vi "Tree.vi"   [LabVIEW 2019, in "DAQmx.lvclass"]
uses:
  DAQmx.lvclass
  C:/Program Files/National Instruments/LabVIEW 2019/vi.lib/JKI/JKI SMO/SMO/SMO.lvclass
  <vilib>/JKI/JKI SMO/SMO/SMO.lvclass
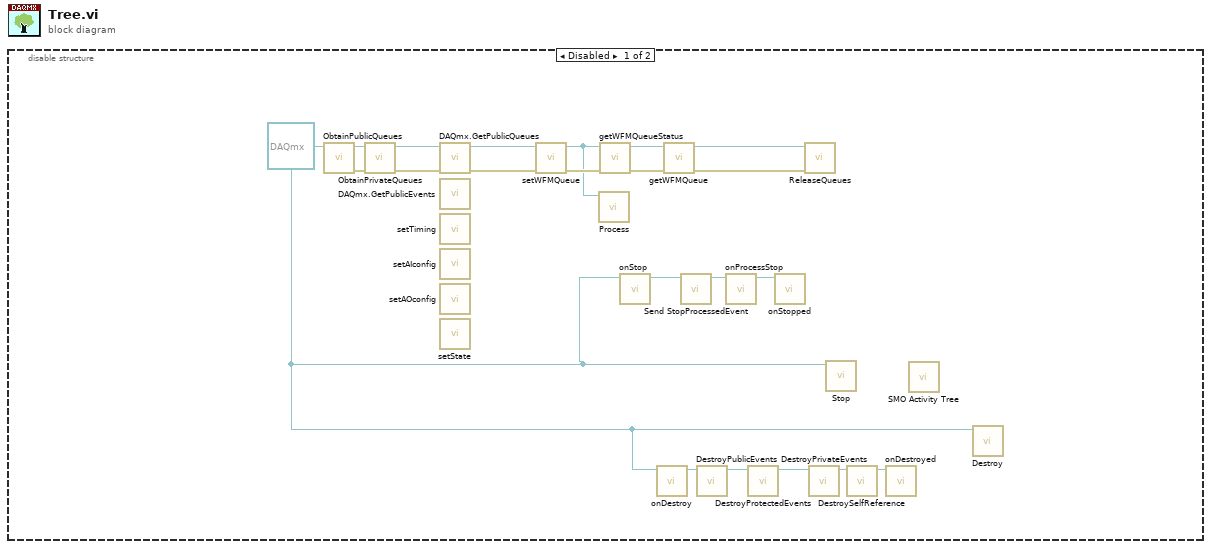
[diagram p0: block diagram]
diagram:
  n1 = disable-structure shown="Disabled" {
    frame Disabled {
      w1 = refnum<class "DAQmx.lvclass"> refnum ("DAQmx")
      n2 = call "ObtainPublicQueues.vi"("DAQmx"=w1) -> ("error out"=w18:errorcluster, "DAQmx out"=w21:refnum<class "DAQmx.lvclass">)  [unwired: 9 in]
      n3 = call "ObtainPrivateQueues.vi"("error in (no error)"=w18, "DAQmx"=w21) -> ("error out"=w17:errorcluster, "DAQmx out"=w20:refnum<class "DAQmx.lvclass">)  [unwired: 8 in]
      n4 = call "DAQmx.GetPublicQueues.vi"("error in (no error)"=w17, "DAQmx"=w20) -> ("error out"=w16:errorcluster, "DAQmx out"=w19:refnum<class "DAQmx.lvclass">)  [unwired: 7 in, 1 out]
      n5 = call "DAQmx.GetPublicEvents.vi"() -> ()  [unwired: 9 in, 3 out]
      n6 = call "setTiming.vi"() -> ()  [unwired: 10 in, 2 out]
      n7 = call "setAIconfig.vi"() -> ()  [unwired: 10 in, 2 out]
      n8 = call "setAOconfig.vi"() -> ()  [unwired: 10 in, 2 out]
      n9 = call "setState.vi"() -> ()  [unwired: 10 in, 2 out]
      n10 = call "setWFMQueue.vi"("error in (no error)"=w16, "DAQmx in"=w19) -> ("error out"=w15:errorcluster, "DAQmx out"=w10:refnum<class "DAQmx.lvclass">)  [unwired: 8 in]
      n11 = call-dynamic "Process.vi"("DAQmx"=w10) -> ()  [unwired: 9 in, 2 out]
      n12 = call "getWFMQueueStatus.vi"("error in (no error)"=w15, "DAQmx in"=w10) -> ("error out"=w13:errorcluster, "DAQmx out"=w14:refnum<class "DAQmx.lvclass">)  [unwired: 6 in, 2 out]
      n13 = call-dynamic "onStop.vi"("SMO"=w1) -> ("SMO out"=w2:refnum<class "DAQmx.lvclass">)  [unwired: 9 in, 1 out]
      n14 = call-dynamic "onDestroy.vi"("DAQmx"=w1) -> ("DAQmx out"=w9:refnum<class "DAQmx.lvclass">)  [unwired: 9 in, 1 out]
      n15 = call "getWFMQueue.vi"("error in (no error)"=w13, "DAQmx in"=w14) -> ("error out"=w11:errorcluster, "DAQmx out"=w12:refnum<class "DAQmx.lvclass">)  [unwired: 7 in, 1 out]
      n16 = call <vilib>:"Send StopProcessedEvent.vi"("SMO"=w2) -> ("SMO out"=w3:refnum<class "DAQmx.lvclass">)  [unwired: 9 in, 1 out]
      n17 = call-dynamic "DestroyPublicEvents.vi"("DAQmx"=w9) -> ("DAQmx out"=w8:refnum<class "DAQmx.lvclass">)  [unwired: 9 in, 1 out]
      n18 = call-dynamic "onProcessStop.vi"("SMO"=w3) -> ("SMO out"=w4:refnum<class "DAQmx.lvclass">)  [unwired: 9 in, 1 out]
      n19 = call-dynamic "DestroyProtectedEvents.vi"("SMO"=w8) -> ("SMO out"=w7:refnum<class "DAQmx.lvclass">)  [unwired: 9 in, 1 out]
      n20 = call-dynamic "onStopped.vi"("SMO"=w4) -> ()  [unwired: 9 in, 2 out]
      n21 = call "ReleaseQueues.vi"("error in (no error)"=w11, "DAQmx"=w12) -> ()  [unwired: 8 in, 2 out]
      n22 = call-dynamic "DestroyPrivateEvents.vi"("DAQmx"=w7) -> ("DAQmx out"=w6:refnum<class "DAQmx.lvclass">)  [unwired: 9 in, 1 out]
      n23 = call <vilib>:"Stop.vi"("SMO"=w1) -> ()  [unwired: 9 in, 2 out]
      n24 = call-dynamic "DestroySelfReference.vi"("SMO"=w6) -> ("SMO out"=w5:refnum<class "DAQmx.lvclass">)  [unwired: 9 in, 1 out]
      n25 = call-dynamic "onDestroyed.vi"("SMO"=w5) -> ()  [unwired: 10 in, 1 out]
      n26 = call <vilib>:"SMO Activity Tree.vi"() -> ()  [unwired: 12 in]
      n27 = call <vilib>:"Destroy.vi"("SMO"=w1) -> ()  [unwired: 10 in, 1 out]
    }
    frame Enabled {
    }
  }
